vi "Waveform - Search.vi"() -> ()   [LabVIEW 2023]
doc: "Shows how to use the Search Waveform VI to find all occurrences of a given search value in a waveform."
panel:
  in  "Tolerance (%)":dbl=10.0
  in  "Search Value":dbl=1.1
  out "Waveform Graph":waveform(dbl)[](graph)
  # "Overview: Demonstrates the use of the Search Waveform VI to detect values within a waveform.\nInstructions:\n1. Specify a Search Value and a Tolerance.\n2. Run the VI. The Fits plot will display the time indices for all values detected within the waveform that match the Search Value within tolerance."
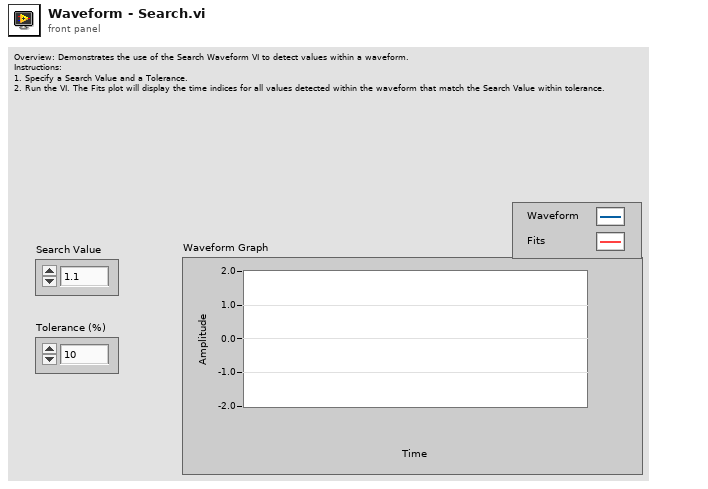
[diagram p1: front panel]
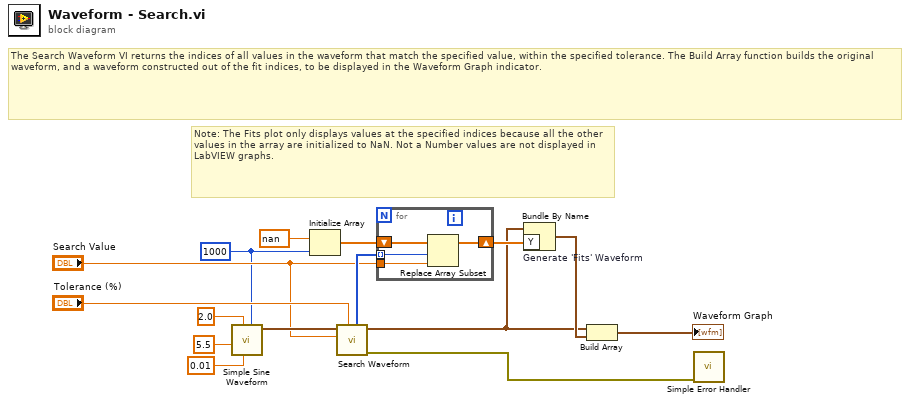
[diagram p0: block diagram]
diagram:
  w5 = 1000 ("n points")
  # "Note: The Fits plot only displays values at the specified indices because all the other values in the array are initialized to NaN. Not a Number values are not displayed in LabVIEW graphs."
  # "The Search Waveform VI returns the indices of all values in the waveform that match the specified value, within the specified tolerance. The Build Array function builds the original waveform, and a waveform constructed out of the fit indices, to be displayed in the Waveform Graph indicator."
  n1 = call "Simple Sine Waveform.vi"("n points"=w5, "delta t"=0.01, "amplitude"=2.0, "n cycles"=5.5 ("frequency")) -> ("sine waveform"=w15:waveform(dbl))  [unwired: 2 in, 5 out]
  n2 = Initialize Array(nan, w5) -> (w3:dbl[])
  n3 = call <vilib>:"Search Waveform.vi"("tolerance (%)"="Tolerance (%)", "value"="Search Value", "waveform in"=w15) -> ("error out"=w1:errorcluster, "waveform out"=w2:waveform(dbl), "indices of fits"=w8:i32[])  [unwired: 2 in, 4 out]
  n4 = for {
    tunnel: w8 -> [w18] mode=indexing
    tunnel: "Search Value" -> [w17]
    shift-right: [w16] -> w6
    shift-left: w3 -> [w19]
    n5 = Replace Array Subset(array=w19, new element=w17, index=w18) -> (w16:dbl[])
  }
  n6 = Bundle By Name "Generate 'Fits' Waveform"(cluster=w2, "Y"=w6) -> (w13:waveform(dbl))
  n7 = Build Array "Build Array"(w2, w13) -> (→"Waveform Graph":waveform(dbl)[])
  n8 = call <vilib>:"Simple Error Handler.vi"("error in (no error)"=w1) -> ()  [unwired: 4 in, 5 out]
